vi "Launcher.vi"() -> ()   [LabVIEW 2021]
uses:
  Root Panel/Root Panel Actor/Root Panel Actor.lvclass
  C:/Users/Thomas/Documents/Projects/TemplateVIEW/Sources/Appearance Actor/Appearance Actor/Appearance Actor.lvclass
  C:/Program Files (x86)/National Instruments/LabVIEW 2021/vi.lib/MGI/Panel Manager/Panel Actor/Panel Actor/Panel Actor.lvclass
  Appearance Actor/Appearance Actor/Appearance Actor.lvclass/Appearance Actor.ctl
  <vilib>/MGI/Panel Manager/Panel/Window Position/Reference Position/Ref Display/Ref Display.lvclass
  C:/Program Files (x86)/National Instruments/LabVIEW 2021/vi.lib/MGI/Panel Manager/Panel/Window Position/Window Position.lvclass
  <vilib>/MGI/Panel Manager/Panel/Window Position/Reference Position/Ref Display/Ref Display.vi
  <vilib>/MGI/Panel Manager/Panel Actor/Panel Actor/Launch Root Panel Window.vi
  <vilib>/MGI/Monitored Actor/Actor Monitor/Actor Monitor/Actor Monitor.lvclass
  <vilib>/MGI/Monitored Actor/Monitored Actor.lvlib
  <vilib>/MGI/Panel Manager/Panel Actor/Panel Actor/Panel Actor.lvclass
  <vilib>/MGI/Panel Manager/Panel/Panel.lvlib
  Appearance Actor/Appearance Actor/Appearance Actor.lvclass
  C:/Program Files (x86)/National Instruments/LabVIEW 2021/vi.lib/MGI/Monitored Actor/Monitored Actor/Monitored Actor/Monitored Actor.lvclass
  C:/Program Files (x86)/National Instruments/LabVIEW 2021/vi.lib/ActorFramework/Actor/Actor.lvclass
  C:/Users/Thomas/Documents/Projects/TemplateVIEW/Sources/Root Panel/Root Panel Actor/Root Panel Actor.lvclass
  C:/Program Files (x86)/National Instruments/LabVIEW 2021/vi.lib/MGI/Panel Manager/Panel/Window Position/Reference Position/Reference Position.lvclass
  C:/Program Files (x86)/National Instruments/LabVIEW 2021/vi.lib/MGI/Panel Manager/Panel/Window Position/Reference Position/Ref Display/Ref Display.lvclass
panel:
  in  "Monitored":bool=TRUE
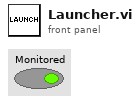
[diagram p1: front panel]
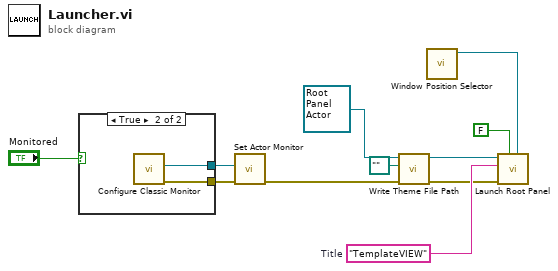
[diagram p0: block diagram]
diagram:
  w7 = "TemplateVIEW"  # Title
  n1 = case shown="True" "Monitored" {
    tunnel: [_ w13] -> w11
    tunnel: [_ w12] -> w10
    frame False {
    }
    frame True {
      n2 = call <vilib>:"Configure Classic Monitor.vi"() -> ("error out"=w12:errorcluster, "Classic Monitor out"=w13:refnum<class "Actor Monitor.lvclass">)  [unwired: 10 in]
    }
  }
  n3 = call <vilib>:"Set Actor Monitor.vi"("error in (no error)"=w10, "Actor Monitor"=w11) -> ("error out"=w3:errorcluster)  [unwired: 9 in]
  n4 = call "Write Theme File Path.vi"("error in (no error)"=w3, "Theme File Path"=path "", "Appearance Actor in"=refnum<class "Root Panel Actor.lvclass"> refnum ("Root Panel.lvlib:Root Panel Actor.lvclass")) -> ("error out"=w2:errorcluster, "Appearance Actor out"=w4:refnum<class "Root Panel Actor.lvclass">)  [unwired: 7 in]
  n5 = call-poly <vilib>:"Window Position Selector.vi"() -> ("Ref Display out"=w8:refnum<class "Ref Display.lvclass">)  [unwired: 10 in, 1 out]
  n6 = call-poly <vilib>:"Launch Root Panel.vi"("Window Position (Maximize First Call)"=w8, "Autoshow? (T)"=FALSE, "Error In"=w2, "Title"=w7, "Panel Actor in"=w4) -> ()  [unwired: 5 in, 2 out]
